vi "complex.vi"() -> ()   [LabVIEW 2013]
panel:
  in  "?":bool
  out "Substraction":dbl
  out "Addition":dbl
  out "Minor":bool
  out "Major":bool
  out "Equal":bool
  out "Divistion":dbl
  out "Multiplication":dbl
  in  "B":dbl
  in  "A":dbl
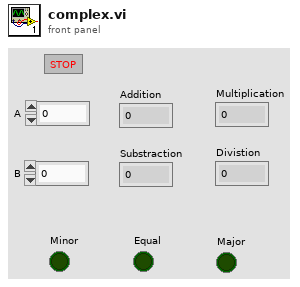
[diagram p1: front panel]
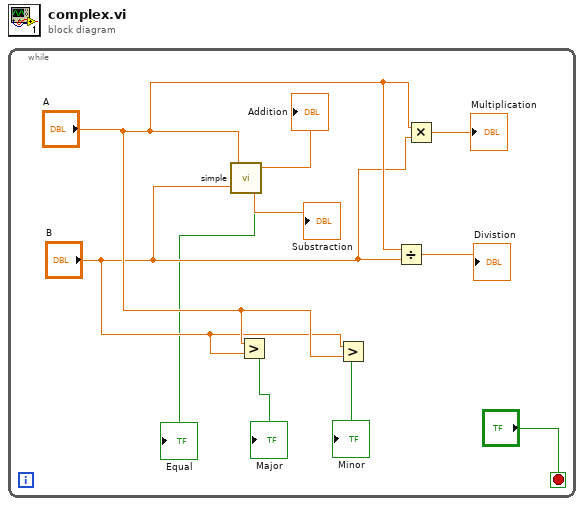
[diagram p0: block diagram]
diagram:
  n1 = while {
    stop <- "?" stop-if-true
    n2 = call "simple.vi"("A"="A", "B"="B") -> ("Addition"=→"Addition":dbl, "Substraction"=→"Substraction":dbl, "Equal"=→"Equal":bool)
    n3 = Greater?(x="A", y="B") -> (0:→"Major":bool)
    n4 = Greater?(x="B", y="A") -> (0:→"Minor":bool)
    n5 = Divide(x="A", y="B") -> (x/y=→"Divistion":dbl)
    n6 = Multiply(x="A", y="B") -> (x*y=→"Multiplication":dbl)
  }
